vi "SimulateMotorPosition.vi"(3 "Reset":bool, 4 "Speed (units/loop)":dbl=50.0, 5 "Goal Position (units)":dbl format="%#_13g") -> (2 "Simulated Position (units)":dbl)   [LabVIEW 2020]
doc: "Simulates a motor position sensor by traveling to the goal angle at a fixed velocity."
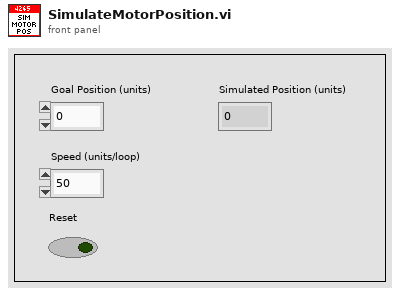
[diagram p1: front panel]
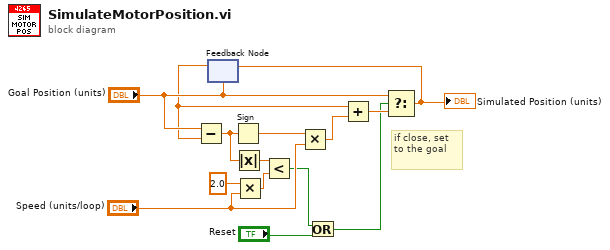
[diagram p0: block diagram]
diagram:
  # "if close, set\nto the goal"
  n1 = feedback #1("Goal Position (units)") -> (w6:dbl)
  n2 = Subtract(x="Goal Position (units)", y=w6) -> (x-y=w7:dbl)
  n3 = Sign(1:w7) -> (0:w4:dbl)
  n4 = Absolute Value(x=w7) -> (abs(x)=w8:dbl)
  n5 = Multiply(x=2.0, y="Speed (units/loop)") -> (x*y=w9:dbl)
  n6 = Less?(x=w8, y=w9) -> (x < y?=w2:bool)
  n7 = Multiply(x=w4, y="Speed (units/loop)") -> (x*y=w5:dbl)
  n8 = Or(x=w2, y="Reset") -> (x .or. y?=w3:bool)
  n9 = Add(x=w6, y=w5) -> (x+y=w12:dbl)
  n10 = Select(t="Goal Position (units)", s=w3, f=w12) -> (s? t:f=w14:dbl)
  "Simulated Position (units)" <- w14
  n11 = feedback-in #1(w14) -> ()
